vi "TTLWaveSubVI.vi"(6 "Error In":errorcluster, 8 "Frequency":dbl, 9 "DC Offset":dbl, 10 "Duty Cycle":dbl, 11 "Amplitude":dbl) -> (0 "Error Out":errorcluster, 3 "Array":dbl[](array[numeric]))   [LabVIEW 2017]
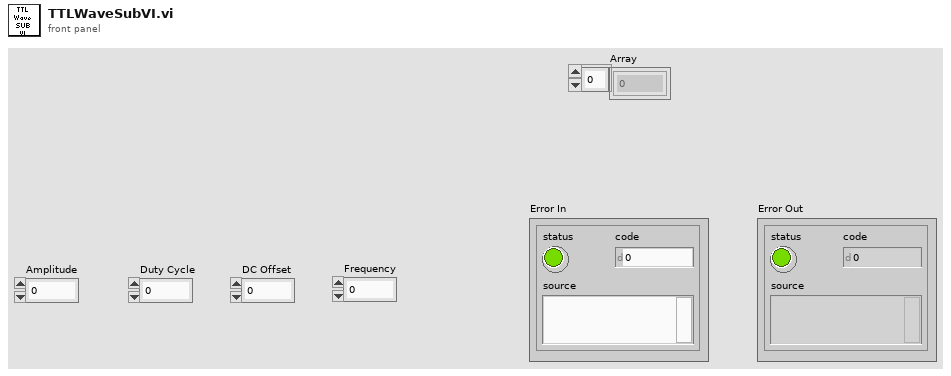
[diagram p1: front panel]
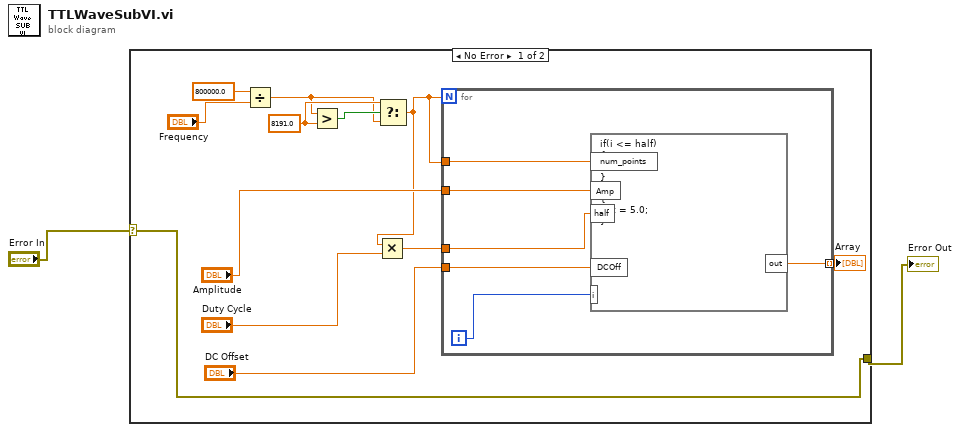
[diagram p0: block diagram]
diagram:
  n1 = case shown="No Error" "Error In" {
    selector: "Error In" -> [w14 w21]
    tunnel: [w14 w21] -> w1
    frame No Error {
      w10 = 8191.0 ("y")
      n2 = Divide(x=800000.0, y="Frequency") -> (x/y=w9:dbl)
      n3 = Greater?(x=w9, y=w10) -> (0:w11:bool)
      n4 = Select(t=w10, s=w11, f=w9) -> (s? t:f=w7:dbl)
      n5 = Multiply(x=w7, y="Duty Cycle") -> (x*y=w6:dbl)
      n6 = for {
        N: w7 -> [_]
        tunnel: w7 -> [w20]
        tunnel: "Amplitude" -> [w19]
        tunnel: w6 -> [w18]
        tunnel: "DC Offset" -> [w16]
        tunnel: [w15] -> w3 mode=indexing
        i -> [w17]
        n7 = formula code="if(i <= half)\n{\nout = 0;\n}\nelse\n{\nout = 5.0;\n}"("num_points"=w20, "Amp"=w19, "half"=w18, "i"=w17, "DCOff"=w16) -> ("out"=w15:dbl)
      }
      "Array" <- w3
    }
    frame Error {
    }
  }
  "Error Out" <- w1
